vi "Configure Trigger.vi"(0 "VISA resource name":refnum<visa-resource-name>, 1 "Delay Method (1: Automatic)":u16(ring)=1 items=["Manual", "Automatic"], 2 "Delay (0)":dbl, 5 "Source (0: Immediate)":u16(ring) items=["Immediate", "Timer", "Manual", "Bus", "External"], 7 "Trigger Timer (0.1)":dbl=0.1, 11 "error in (no error)":errorcluster, 12 "Trigger Count Method (0: Manual)":u16(ring) items=["Manual", "Infinity"], 13 "Trigger Count (1)":i32=1) -> (4 "VISA resource name out":refnum<visa-resource-name>, 15 "error out":errorcluster)   [LabVIEW 2020, in "Keithley 27XX.lvlib"]
doc: "This VI allows you to configure the triggering for the multimeter. It contains setting for which type of trigger to setup, as well as settings which are specific to each type of trigger."
uses:
  <instrlib>/Keithley 27XX/Keithley 27XX.lvlib
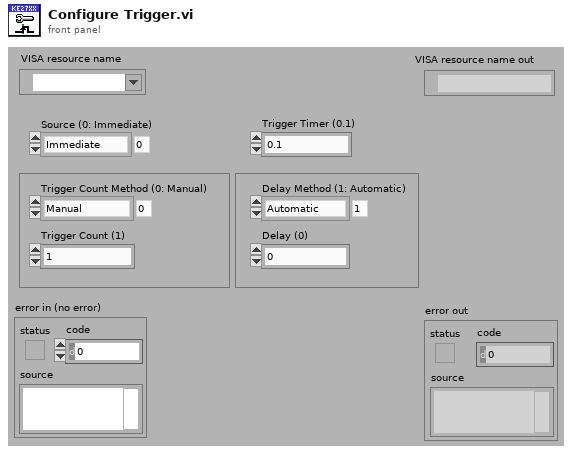
[diagram p1: front panel]
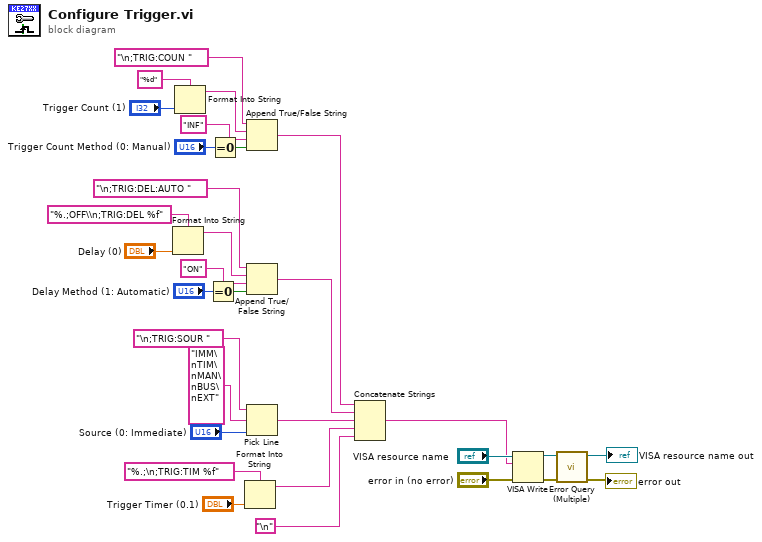
[diagram p0: block diagram]
diagram:
  n1 = Format Into String(format string="%.;OFF\\n;TRIG:DEL %f" ("string (\"\")"), "Delay (0)") -> (resulting string=w13:string)  [unwired: 2 in, 1 out]
  n2 = Format Into String(format string="%d" ("string (\"\")"), "Trigger Count (1)") -> (resulting string=w10:string)  [unwired: 2 in, 1 out]
  n3 = Equal To 0?(x="Delay Method (1: Automatic)") -> (x = 0?=w27:bool)
  n4 = Equal To 0?(x="Trigger Count Method (0: Manual)") -> (x = 0?=w30:bool)
  n5 = Format Into String(format string="%.;\n;TRIG:TIM %f" ("initial string"), "Trigger Timer (0.1)") -> (resulting string=w2:string)  [unwired: 2 in, 1 out]
  n6 = Append True/False String(1:w30, 2:"INF" ("string (\"\")"), 3:w10, 4:"\n;TRIG:COUN " ("string (\"\")")) -> (0:w5:string)
  n7 = Append True/False String(1:w27, 2:"ON" ("string (\"\")"), 3:w13, 4:"\n;TRIG:DEL:AUTO " ("string (\"\")")) -> (0:w4:string)
  n8 = Pick Line(string ("")="\n;TRIG:SOUR ", multi-line string="IMM\nTIM\nMAN\nBUS\nEXT" ("string (\"\")"), line index="Source (0: Immediate)") -> (output string=w3:string)
  n9 = Concatenate Strings(w5, w4, w3, w2, "\n") -> (w18:string)
  n10 = VISA Write(VISA resource name="VISA resource name", write buffer=w18, error in (no error)="error in (no error)") -> (VISA resource name out=w9:refnum<visa-resource-name>, error out=w8:errorcluster)  [unwired: 1 out]
  n11 = call <instrlib>:"Error Query (Multiple).vi"("VISA resource name"=w9, "error in (no error)"=w8) -> ("VISA resource name out"=→"VISA resource name out":refnum<visa-resource-name>, "error out"=→"error out":errorcluster)  [unwired: 10 in, 2 out]
